vi "4021_output.vi"(0 "Address":T1, 2 "Function":T2, 3 "Set to:":dbl min=0.0 max=20.0 format="%.3f", 4 "Channel Name":string) -> (5 "Comment":string, 7 "Reading":dbl format="%.3f")   [LabVIEW 2018]
uses:
  ADAM Client/Sub VIs/ADAM Controls/Function_ADAM.ctl
  ADAM Client/Sub VIs/ADAM Controls/Address.ctl
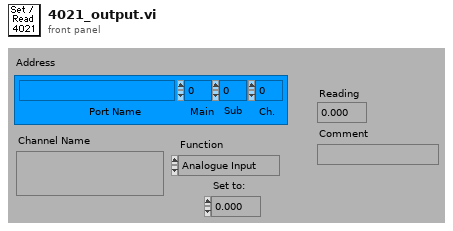
[diagram p1: front panel]
types:
  T1 = typedef "Address.ctl" = cluster{"Main":i32, "Ch.":i32, "Sub":i32, "Port Name":string}
  T2 = typedef "Function_ADAM.ctl" = enum16{"Analogue Input", "Digital Input", "Event counter", "Event rate", "Analogue Output", "Digital Output", "Relay Output"}
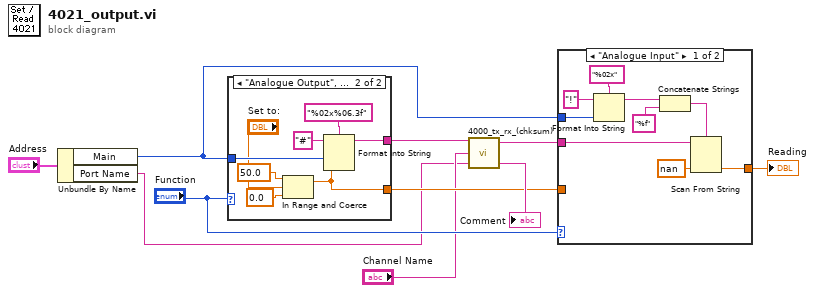
[diagram p0: block diagram]
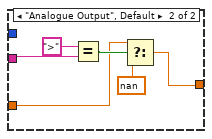
[diagram p2: hidden frame]
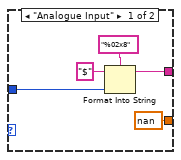
[diagram p3: hidden frame]
diagram:
  n1 = Unbundle By Name("Address") -> ("Main"=w2:i32, "Port Name"=w1:string)
  n2 = case shown="\"Analogue Output\", Default" "Function" {
    tunnel: [w13 w21] -> w8
    tunnel: w2 -> [w12 w20]
    tunnel: [nan ("Set to:") w16] -> w5
    frame "Analogue Input" {
      n3 = Format Into String(format string="%02x8", initial string="$", w12) -> (resulting string=w13:string)  [unwired: 1 in, 1 out]
    }
    frame "Analogue Output", Default {
      n4 = In Range and Coerce(upper limit=50.0 ("Max"), x="Set to:", lower limit=0.0 ("Min")) -> (coerced(x)=w16:dbl)  [unwired: 1 out]
      n5 = Format Into String(format string="%02x%06.3f", initial string="#", w20, w16) -> (resulting string=w21:string)  [unwired: 1 in, 1 out]
    }
  }
  n6 = call "4000_tx_rx_(chksum).vi"("Write String"=w8, "Channel Name"="Channel Name", "Port Name"=w1) -> ("Read"=w7:string, "Comment out"=→"Comment":string)  [unwired: 2 in, 1 out]
  n7 = case shown="\"Analogue Input\"" "Function" {
    tunnel: [w32 w35] -> w9
    tunnel: w2 -> [w28 _]
    tunnel: w7 -> [w24 w38]
    tunnel: w5 -> [_ w34]
    frame "Analogue Input" {
      n8 = Format Into String(format string="%02x", initial string="!", w28) -> (resulting string=w26:string)  [unwired: 1 in, 1 out]
      n9 = Concatenate Strings(w26, "%f") -> (w27:string)
      n10 = Scan From String(format string=w27, input string=w24, default 1=nan ("Reading")) -> (output 1=w32:dbl)  [unwired: 2 in, 3 out]
    }
    frame "Analogue Output", Default {
      n11 = Equal?(x=">", y=w38) -> (x = y?=w36:bool)
      n12 = Select(t=w34, s=w36, f=nan) -> (s? t:f=w35:dbl)
    }
  }
  "Reading" <- w9
